vi "Convert Number to Fault.vi"(11 "Number":i32) -> (3 "Fault":T1=enum."Motor Stall")   [LabVIEW 2018, in "Mock Pump Controller.lvlib"]
uses:
  Mock Pump Controller.lvlib
  Typedefs/Faults.ctl
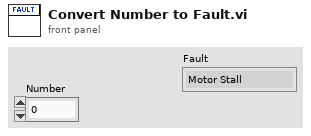
[diagram p1: front panel]
types:
  T1 = typedef "Mock Pump Controller.lvlib/Faults.ctl" = enum16{"Upper Pressure Fault", "Lower Pressure Fault", "Motor Stall"}
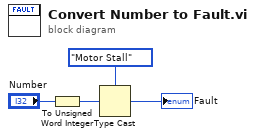
[diagram p0: block diagram]
diagram:
  n1 = To Unsigned Word Integer(number="Number") -> (unsigned 16bit integer=w2:u16)
  n2 = Type Cast(type=Faults."Motor Stall" ("Faults (enum)"), x=w2) -> (*(type *) &x=→"Fault":T1)
